vi "TuningParams.vi"(11 "RHB Version":T1) -> (0 "LY Gradient":dbl, 1 "LX Gradient":dbl, 2 "RY Gradient":dbl, 3 "RX Gradient":dbl, 4 "Right Poti Offset":dbl, 5 "Left Poti Offset":dbl, 6 "Right Poti Gradient":dbl, 7 "Left Poti Gradient":dbl)   [LabVIEW 2019]
uses:
  TypeDefs/ReHandyBotVersion.ctl
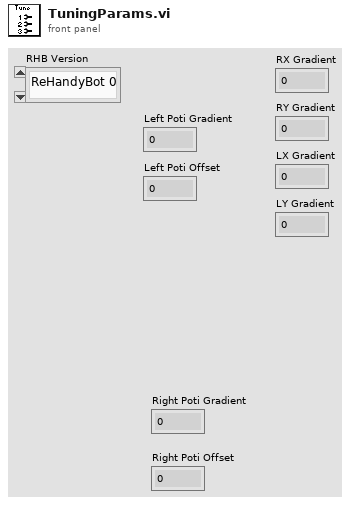
[diagram p1: front panel]
types:
  T1 = typedef "ReHandyBotVersion.ctl" = enum16{"ReHandyBot 0", "ReHandyBot 1", "ReHandyBot 2", "ReHandyBot 3"}
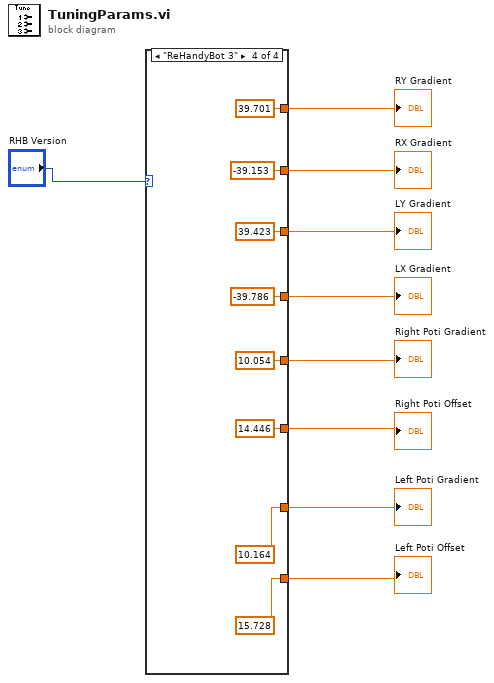
[diagram p0: block diagram]
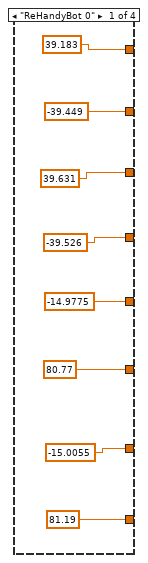
[diagram p2: hidden frame]
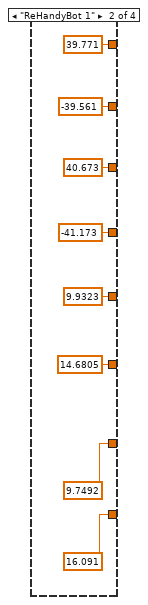
[diagram p3: hidden frame]
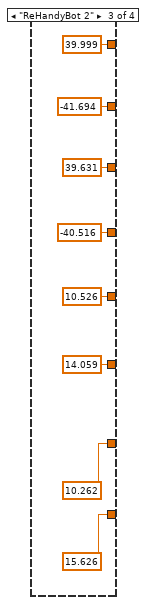
[diagram p4: hidden frame]
diagram:
  n1 = case shown="\"ReHandyBot 3\"" "RHB Version" {
    tunnel: [39.183 39.771 39.999 39.701] -> w2
    tunnel: [-39.449 -39.561 -41.694 -39.153] -> w3
    tunnel: [39.631 40.673 39.631 39.423] -> w4
    tunnel: [-39.526 -41.173 -40.516 -39.786] -> w5
    tunnel: [-14.9775 9.9323 10.526 10.054] -> w6
    tunnel: [80.77 14.6805 14.059 14.446] -> w7
    tunnel: [-15.0055 9.7492 10.262 10.164] -> w8
    tunnel: [81.19 16.091 15.626 15.728] -> w9
    frame "ReHandyBot 0" {
    }
    frame "ReHandyBot 1" {
    }
    frame "ReHandyBot 2" {
    }
    frame "ReHandyBot 3" {
    }
  }
  "Left Poti Offset" <- w9
  "Left Poti Gradient" <- w8
  "Right Poti Offset" <- w7
  "Right Poti Gradient" <- w6
  "LX Gradient" <- w5
  "LY Gradient" <- w4
  "RX Gradient" <- w3
  "RY Gradient" <- w2
